vi "截图保存.vi"() -> ()   [LabVIEW 2013]
uses:
  <vilib>/printing/EasyPrintingControls.llb/contents.ctl
  <vilib>/printing/EasyPrintingControls.llb/report_type.ctl
  <vilib>/Utility/NIReport.llb/NI_report.lvclass
  <vilib>/printing/EasyPrinting.llb/Easy Print VI Panel or Documentation (path).vi
  <vilib>/Utility/NIReport.llb/NI_ReportGenerationCore.lvlib
panel:
  out "路径 2":path
  out "路径":path
  in  "产品ID":string="XX"
  out "error out":errorcluster caption="错误输出"
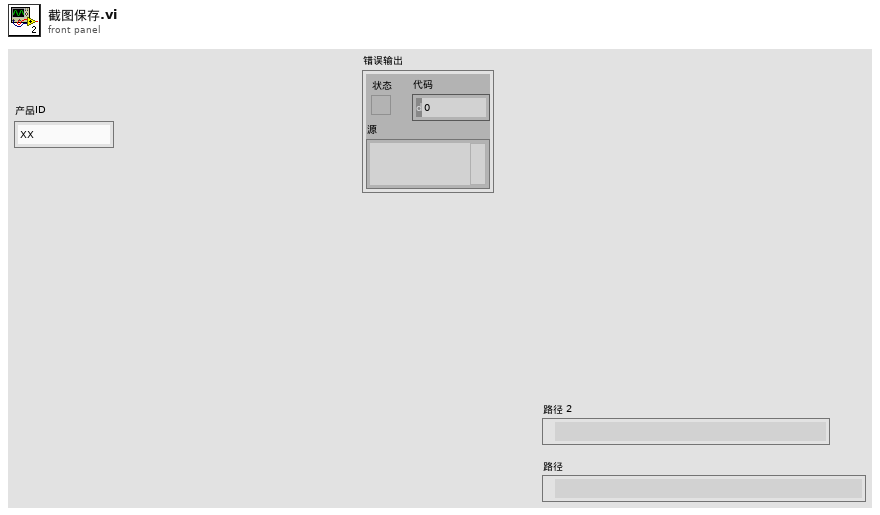
[diagram p1: front panel]
types:
  T1 = typedef "NI_ReportGenerationCore.lvlib/report_type.ctl" = u16
  T2 = typedef "NI_ReportGenerationCore.lvlib/contents.ctl" = u16
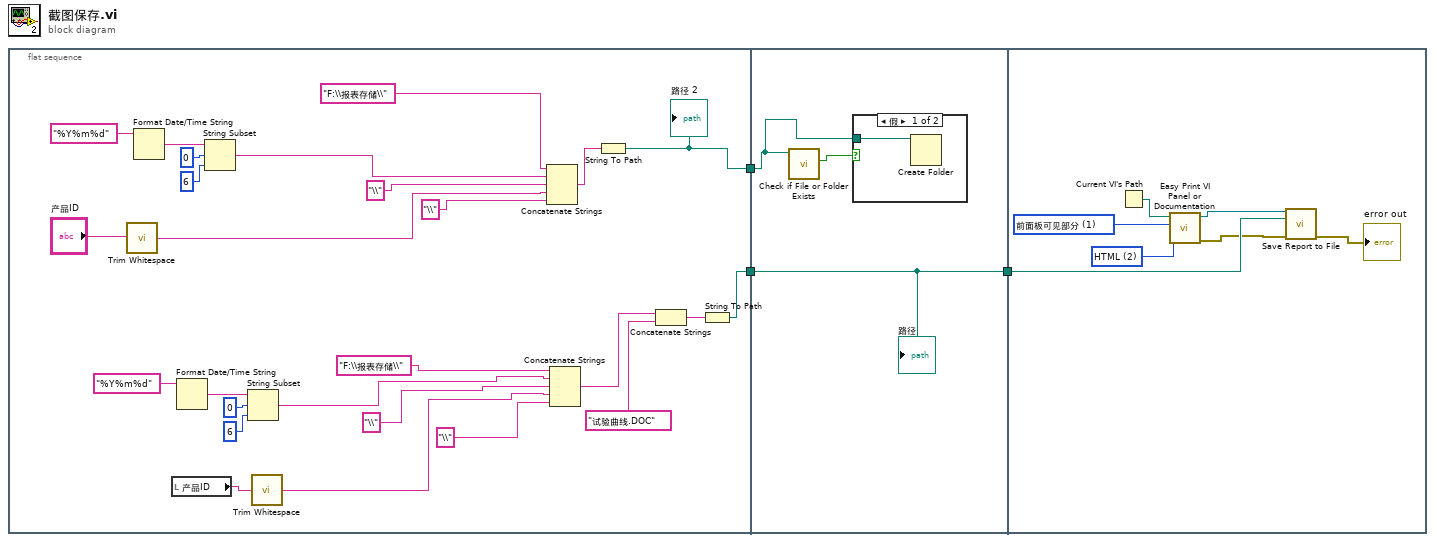
[diagram p0: block diagram]
diagram:
  n1 = flat-sequence {
    tunnel: [w15] -> w3
    tunnel: [w4] -> w1
    tunnel: w3 -> [w31]
    tunnel: [w30] -> w2
    tunnel: w1 -> [w30]
    tunnel: w2 -> [w40]
    frame #0 {
      n2 = call <vilib>:"Trim Whitespace.vi"("string"="产品ID") -> ("trimmed string"=w17:string)  [unwired: 1 in]
      n3 = Format Date/Time String(time format string (%c)="%Y%m%d" ("时间格式字符串(%c)")) -> (date/time string=w26:string)  [unwired: 2 in]
      n4 = local read "产品ID"() -> (w7:string)
      n5 = Format Date/Time String(time format string (%c)="%Y%m%d" ("时间格式字符串(%c)")) -> (date/time string=w14:string)  [unwired: 2 in]
      n6 = String Subset(string=w26, offset (0)=0 ("偏移量(0)"), length (rest)=6 ("长度（剩余）")) -> (substring=w19:string)
      n7 = String Subset(string=w14, offset (0)=0 ("偏移量(0)"), length (rest)=6 ("长度（剩余）")) -> (substring=w9:string)
      n8 = call <vilib>:"Trim Whitespace.vi"("string"=w7) -> ("trimmed string"=w6:string)  [unwired: 1 in]
      n9 = Concatenate Strings("F:\\报表存储\\" ("字符串"), w19, "\\" ("字符串"), w17, "\\" ("字符串")) -> (w25:string)
      n10 = Concatenate Strings("F:\\报表存储\\" ("字符串"), w9, "\\" ("字符串"), w6, "\\" ("字符串")) -> (w22:string)
      n11 = String To Path(string=w25) -> (path=w15:path)
      "路径 2" <- w15
      n12 = Concatenate Strings(w22, "试验曲线.DOC" ("字符串")) -> (w23:string)
      n13 = String To Path(string=w23) -> (path=w4:path)
    }
    frame #1 {
      n14 = call <vilib>:"Check if File or Folder Exists.vi"("path"=w31) -> ("file or folder exists?"=w32:bool)  [unwired: 8 in, 2 out]
      n15 = case shown="假" w32 {
        tunnel: w31 -> [w33 _]
        frame False {
          n16 = Create Folder(path (use dialog)=w33) -> ()  [unwired: 2 in, 3 out]
        }
        frame True {
        }
      }
      "路径" <- w30
    }
    frame #2 {
      w36 = T1 2 items=["快速打印", "标准报表", "HTML", "双字节", "Excel"] ("report type (Quick Print)")
      w37 = T2 1 items=["完整前面板", "前面板可见部分", "图标、说明、前面板和程序框图", "说明信息: 使用前面板", "说明信息: 作为子VI使用", "说明信息: 完整", "说明信息: 自定义"] ("contents (complete front panel)")
      n17 = Current VI's Path() -> (path=w38:path)
      n18 = call-poly <vilib>:"Easy Print VI Panel or Documentation.vi"("report type (Quick Print)"=w36, "contents (complete front panel)"=w37, "VI path"=w38) -> ("error out"=w34:errorcluster, "report out"=w35:refnum<class "NI_report.lvclass">)  [unwired: 1 in, 6 out]
      n19 = call-dynamic "Save Report to File.vi"("report in"=w35, "report file path"=w40, "error in (no error)"=w34) -> ("error out"=→"error out":errorcluster)  [unwired: 2 in, 10 out]
    }
  }
